vi "Periodic Tasks.vi"(8 "error in":errorcluster) -> ()   [LabVIEW 2016]
doc: "This VI runs in parallel to other tasks. It can contain as many user-defined periodic loops as you need. These can carry out PID or other sorts of timed response."
uses:
  <vilib>/Rock Robotics/WPI/DriverStation/WPI_DriverStationRobotMode2.ctl
  Autonomous VIs/Autonomous Commands/Autonomous Command Names.ctl
  Autonomous VIs/Autonomous Exec/Autonomous Play Definition.ctl
  <vilib>/Rock Robotics/Network Tables/NT Write String Array.vi
  Global Variables/File Path Globals.vi
  Robot Global Data.vi
  <vilib>/Rock Robotics/Network Tables/NT Write String.vi
  Global Variables/Autonomous Exec Info.vi
  <vilib>/Rock Robotics/Network Tables/SD Read String.vi
  Global Variables/Folder Names.vi
  Global Variables/Refnum Names.vi
  <vilib>/Rock Robotics/WPI/Utilities/WPI_GetSetVariantRefNum.vi
  Global Variables/Sensor Data.vi
  Global Variables/Auto Drive Calibrations.vi
panel:
  out "Waveform Chart":T1(graph)
  out "error out":errorcluster
  out "File Name of Play":string
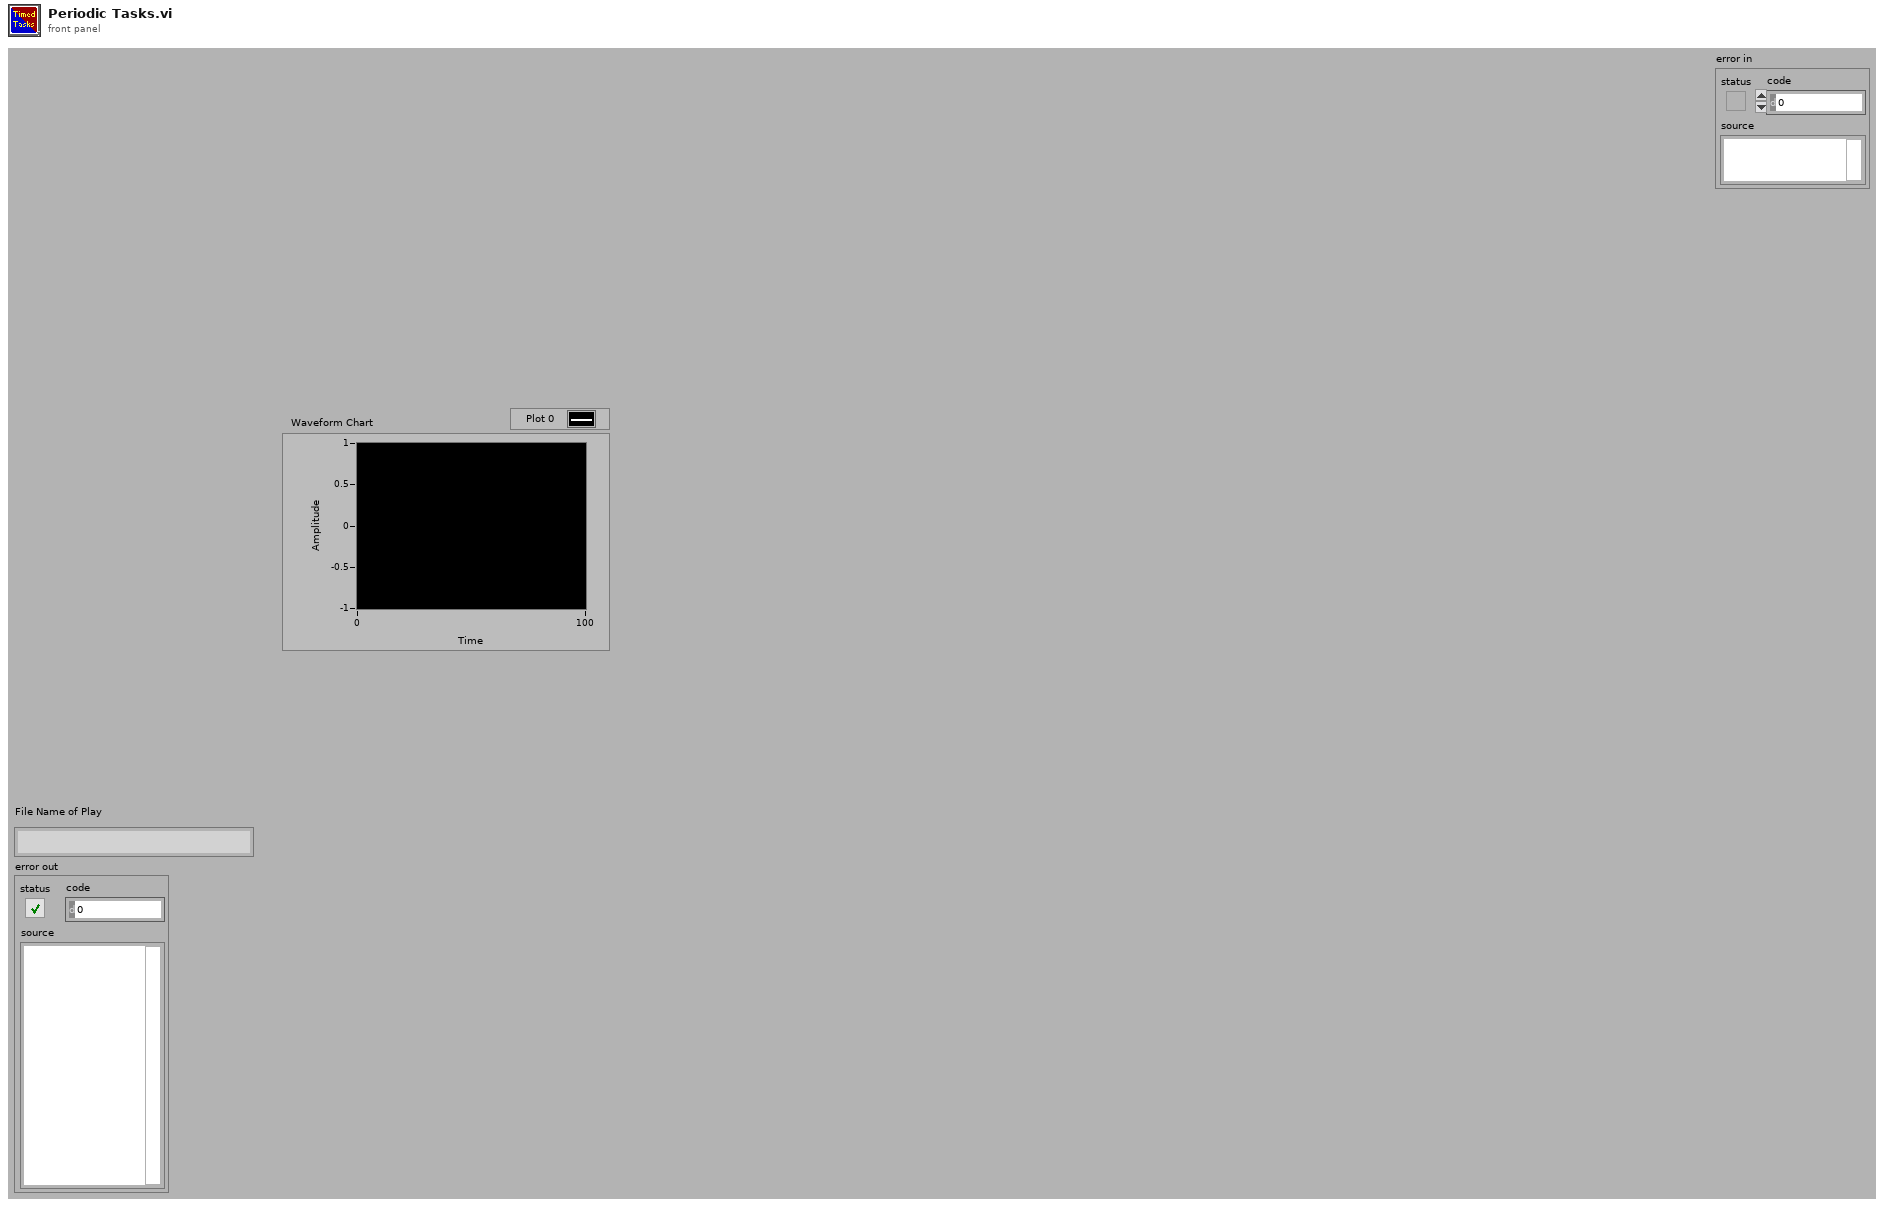
[diagram p1: front panel]
types:
  T1 = cluster{"Goal":dbl, "Process Variable":dbl, "Max Ouput":dbl, dbl, dbl, dbl, dbl}
  T2 = typedef "WPI_DriverStationRobotMode2.ctl" = enum16{"Autonomous Disabled", "Autonomous Enabled", "Teleop Disabled", "Teleop Enabled", "Disconnected", "Finish", "Test Disabled", "Test Enabled", "Emergency Stopped"}
  T3 = typedef "Autonomous Command Names.ctl" = enum16{"No Op", "Command Drive+Climb Shift", "Command Wait", "Command Deliver Gear", "Command Buffer", "Command Drive Path", "Command Drive Time", "Command Shoot", "Command Turn to Heading", "Command Run Conveyor", "Command Spinup Shooter", "Command Deliver Gear Front", "Command Toggle Intake Rotation", "DO NOT USE", "Command Agitate Hopper", "Command Pre-Buffer", "Command Turn to Target", "Command Deliver Gear with Safety", "Command Drive Time with IMU", "Command Drive to Encoders"}
  T4 = typedef "Autonomous Play Definition.ctl" = cluster{"Play Name":string, "Command List":cluster{"Param 1":dbl, "Param 2":dbl, "Autonomous Command Name":T3, "Concurrent":bool, "Param 3":dbl, "Param 4":string}[], "Play Description":string}
  T5 = cluster{"Param 1":dbl, "Param 2":dbl, "Autonomous Command Name":T3, "Concurrent":bool, "Param 3":dbl, "Param 4":string}[]
  T6 = cluster{"Param 1":dbl, "Param 2":dbl, "Autonomous Command Name":T3, "Concurrent":bool, "Param 3":dbl, "Param 4":string}
  T7 = typedef "WPI_JoystickDevRef.ctl" = cluster{"Device":T8}
  T8 = typedef "WPI_JoystickDeviceEnum.ctl" = enum16{"USB 0", "USB 1", "USB 2", "USB 3", "USB 4", "USB 5"}
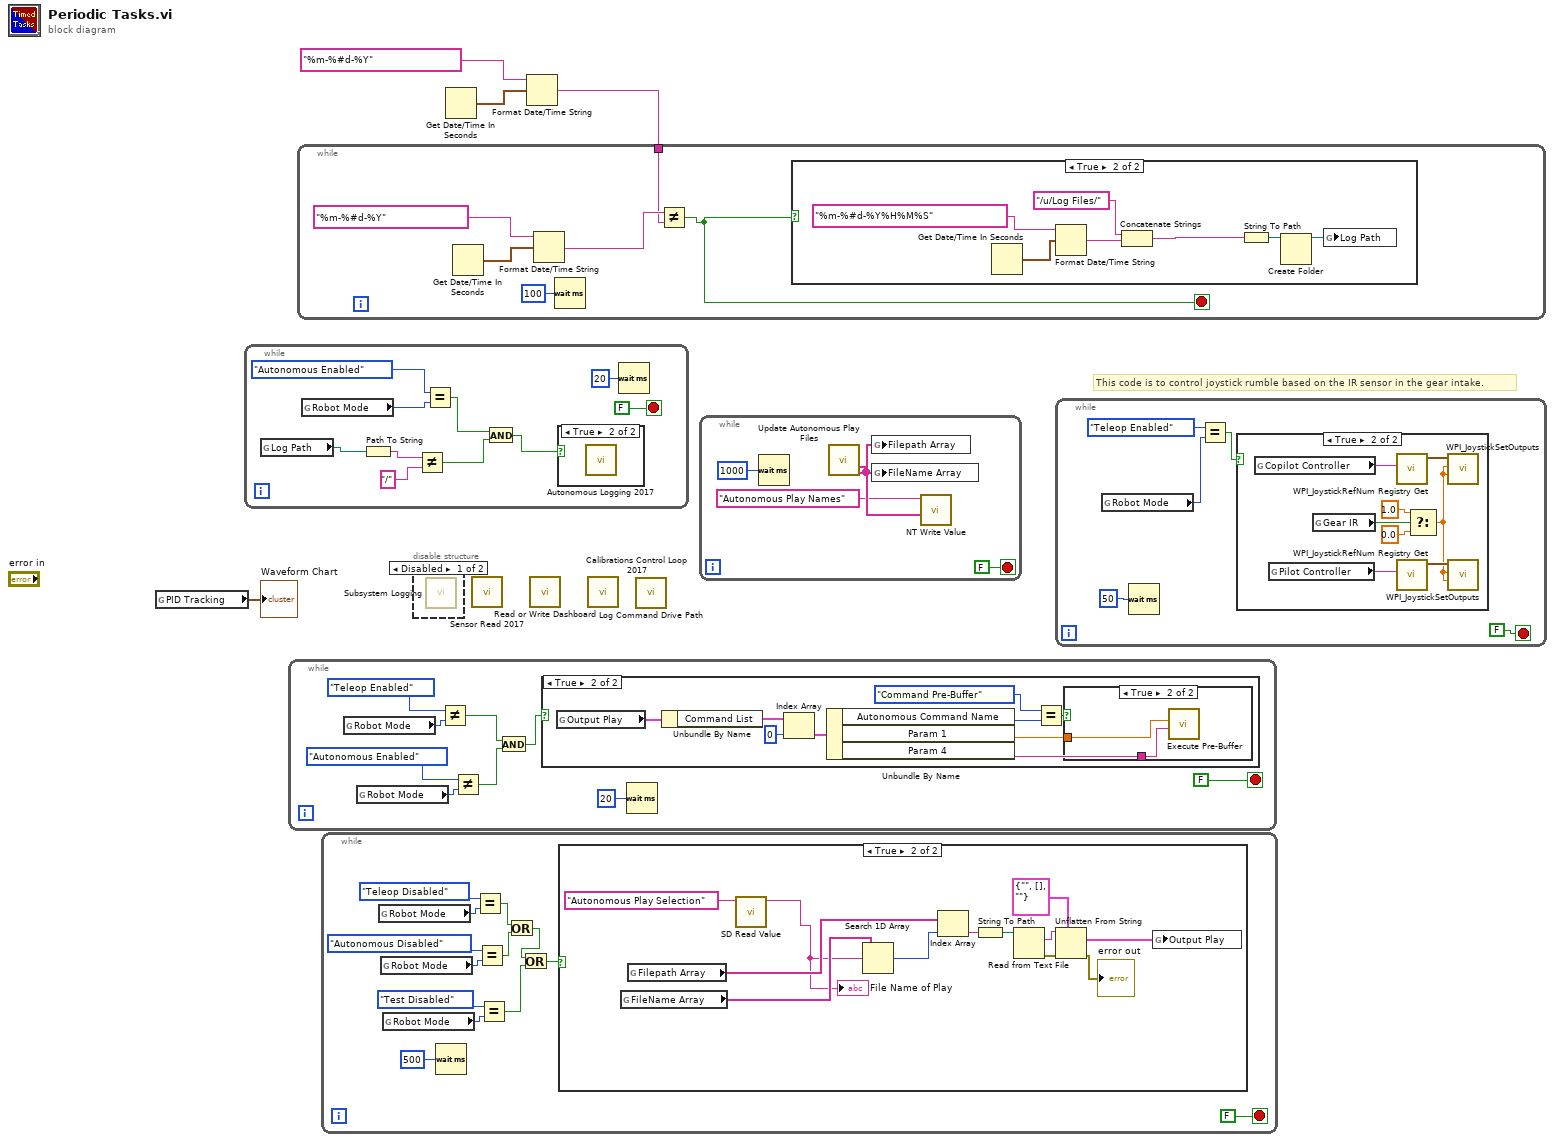
[diagram p0: block diagram]
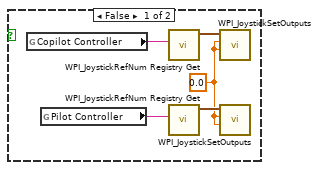
[diagram p3: hidden frame]
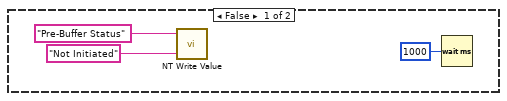
[diagram p7: hidden frame]
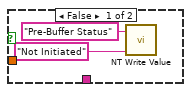
[diagram p8: hidden frame]
diagram:
  # "This code is to control joystick rumble based on the IR sensor in the gear intake."
  n1 = global read "Auto Drive Calibrations.vi" "PID Tracking"() -> (→"Waveform Chart":T1)
  n2 = while {
    stop <- FALSE stop-if-true
    n3 = global read "Folder Names.vi" "Log Path"() -> (w10:path)
    n4 = global read "Robot Global Data.vi" "Robot Mode"() -> (w13:T2)
    n5 = Path To String(path=w10) -> (string=w9:string)
    n6 = Not Equal?(x=w9, y="/") -> (x != y?=w5:bool)
    n7 = Equal?(x=WPI_DriverStationRobotMode2."Autonomous Enabled", y=w13) -> (x = y?=w6:bool)
    n8 = And(x=w6, y=w5) -> (x .and. y?=w7:bool)
    n9 = case shown="True" w7 {
      frame False {
      }
      frame True {
        n10 = call "Autonomous Logging 2017.vi"() -> ()  [unwired: 12 in]
      }
    }
    n11 = Wait (ms)(milliseconds to wait=u32 20) -> ()  [unwired: 1 out]
  }
  n12 = while {
    stop <- FALSE stop-if-true
    n13 = global read "Robot Global Data.vi" "Robot Mode"() -> (w21:T2)
    n14 = global read "Robot Global Data.vi" "Robot Mode"() -> (w19:T2)
    n15 = Not Equal?(x=WPI_DriverStationRobotMode2."Teleop Enabled", y=w21) -> (x != y?=w16:bool)
    n16 = Not Equal?(x=WPI_DriverStationRobotMode2."Autonomous Enabled", y=w19) -> (x != y?=w17:bool)
    n17 = And(x=w16, y=w17) -> (x .and. y?=w15:bool)
    n18 = case shown="True" w15 {
      frame False {
        n19 = call-poly <vilib>:"NT Write Value.vi"("String"="Not Initiated", "Name"="Pre-Buffer Status") -> ()  [unwired: 9 in, 1 out]
        n20 = Wait (ms)(milliseconds to wait=u32 1000) -> ()  [unwired: 1 out]
      }
      frame True {
        n21 = global read "Autonomous Exec Info.vi" "Output Play"() -> (w35:T4)
        n22 = Unbundle By Name(w35) -> ("Command List"=w34:T5)
        n23 = Index Array(array=w34, index=0) -> (element=w32:T6)
        n24 = Unbundle By Name(w32) -> ("Autonomous Command Name"=w31:T3, "Param 1"=w28:dbl, "Param 4"=w27:string)
        n25 = Equal?(x=Autonomous_Command_Names."Command Pre-Buffer", y=w31) -> (x = y?=w29:bool)
        n26 = case shown="True" w29 {
          tunnel: w28 -> [_ w39]
          tunnel: w27 -> [_ w38]
          frame False {
            n27 = call-poly <vilib>:"NT Write Value.vi"("String"="Not Initiated", "Name"="Pre-Buffer Status") -> ()  [unwired: 9 in, 1 out]
          }
          frame True {
            n28 = call "Execute Pre-Buffer.vi"("MP Name"=w38, "PIDF Profile Slot Select"=w39) -> ()  [unwired: 10 in]
          }
        }
      }
    }
    n29 = Wait (ms)(milliseconds to wait=u32 20) -> ()  [unwired: 1 out]
  }
  n30 = while {
    stop <- FALSE stop-if-true
    n31 = global read "Robot Global Data.vi" "Robot Mode"() -> (w51:T2)
    n32 = global read "Robot Global Data.vi" "Robot Mode"() -> (w49:T2)
    n33 = global read "Robot Global Data.vi" "Robot Mode"() -> (w47:T2)
    n34 = Wait (ms)(milliseconds to wait=u32 500) -> ()  [unwired: 1 out]
    n35 = Equal?(x=WPI_DriverStationRobotMode2."Teleop Disabled", y=w51) -> (x = y?=w46:bool)
    n36 = Equal?(x=WPI_DriverStationRobotMode2."Autonomous Disabled", y=w49) -> (x = y?=w45:bool)
    n37 = Equal?(x=WPI_DriverStationRobotMode2."Test Disabled", y=w47) -> (x = y?=w42:bool)
    n38 = Or(x=w46, y=w45) -> (x .or. y?=w43:bool)
    n39 = Or(x=w43, y=w42) -> (x .or. y?=w44:bool)
    n40 = case shown="True" w44 {
      frame False {
      }
      frame True {
        n41 = global read "File Path Globals.vi" "FileName Array"() -> (w64:string[])
        n42 = global read "File Path Globals.vi" "Filepath Array"() -> (w63:string[])
        n43 = call-poly <vilib>:"SD Read Value.vi"("Name"="Autonomous Play Selection") -> ("String"=w55:string)  [unwired: 8 in, 2 out]
        "File Name of Play" <- w55
        n44 = Search 1D Array(1D array=w64, element=w55) -> (index of element=w62:i32)  [unwired: 1 in]
        n45 = Index Array(array=w63, index=w62) -> (element=w61:string)
        n46 = String To Path(string=w61) -> (path=w57:path)
        n47 = Read from Text File(file (use dialog)=w57) -> (text=w60:string, error out=w58:errorcluster)  [unwired: 3 in, 2 out]
        n48 = Unflatten From String(type=T4 {"Play Name"="", "Command List"=[], "Play Description"=""}, binary string=w60, error in (no error)=w58) -> (value=w53:T4, error out=→"error out":errorcluster)  [unwired: 2 in, 1 out]
        n49 = global write "Autonomous Exec Info.vi" "Output Play"(w53) -> ()
      }
    }
  }
  n50 = disable-structure shown="Disabled" {
    frame Disabled {
      n51 = call "Subsystem Logging.vi"() -> ()  [unwired: 12 in]
    }
    frame Enabled {
    }
  }
  n52 = Get Date/Time In Seconds() -> (seconds since 1Jan1904=w3:timestamp)
  n53 = call "Sensor Read 2017.vi"() -> ()  [unwired: 12 in]
  n54 = Format Date/Time String(time format string (%c)="%m-%#d-%Y", seconds (now)=w3) -> (date/time string=w2:string)  [unwired: 1 in]
  n55 = while {
    tunnel: w2 -> [w66]
    stop <- w65 stop-if-true
    n56 = Get Date/Time In Seconds() -> (seconds since 1Jan1904=w70:timestamp)
    n57 = Format Date/Time String(time format string (%c)="%m-%#d-%Y", seconds (now)=w70) -> (date/time string=w67:string)  [unwired: 1 in]
    n58 = Wait (ms)(milliseconds to wait=u32 100) -> ()  [unwired: 1 out]
    n59 = Not Equal?(x=w67, y=w66) -> (x != y?=w65:bool)
    n60 = case shown="True" w65 {
      frame False {
      }
      frame True {
        n61 = Get Date/Time In Seconds() -> (seconds since 1Jan1904=w77:timestamp)
        n62 = Format Date/Time String(time format string (%c)="%m-%#d-%Y%H%M%S", seconds (now)=w77) -> (date/time string=w75:string)  [unwired: 1 in]
        n63 = Concatenate Strings("/u/Log Files/" ("string"), w75) -> (w74:string)
        n64 = String To Path(string=w74) -> (path=w73:path)
        n65 = Create Folder(path (use dialog)=w73) -> (created path=w72:path)  [unwired: 2 in, 2 out]
        n66 = global write "Folder Names.vi" "Log Path"(w72) -> ()
      }
    }
  }
  n67 = call "Read or Write Dashboard.vi"() -> ()  [unwired: 12 in]
  n68 = call "Calibrations Control Loop 2017.vi"() -> ()  [unwired: 12 in]
  n69 = call "Log Command Drive Path.vi"() -> ()  [unwired: 12 in]
  n70 = while {
    stop <- FALSE stop-if-true
    n71 = Wait (ms)(milliseconds to wait=u32 1000) -> ()  [unwired: 1 out]
    n72 = call "Update Autonomous Play Files.vi"() -> ("Filepath Array"=w80:string[], "filename array"=w79:string[])  [unwired: 12 in, 2 out]
    n73 = global write "File Path Globals.vi" "Filepath Array"(w80) -> ()
    n74 = global write "File Path Globals.vi" "FileName Array"(w79) -> ()
    n75 = call-poly <vilib>:"NT Write Value.vi"("String Array"=w79, "Name"="Autonomous Play Names") -> ()  [unwired: 9 in, 1 out]
  }
  n76 = while {
    stop <- FALSE stop-if-true
    n77 = global read "Robot Global Data.vi" "Robot Mode"() -> (w83:T2)
    n78 = Wait (ms)(milliseconds to wait=u32 50) -> ()  [unwired: 1 out]
    n79 = Equal?(x=WPI_DriverStationRobotMode2."Teleop Enabled", y=w83) -> (x = y?=w84:bool)
    n80 = case shown="True" w84 {
      frame False {
        w90 = 0.0
        n81 = global read "Refnum Names.vi" "Copilot Controller"() -> (w88:string)
        n82 = global read "Refnum Names.vi" "Pilot Controller"() -> (w89:string)
        n83 = call <vilib>:"WPI_JoystickRefNum Registry Get.vi"("refnum name"=w88) -> ("JoystickDevRef"=w92:T7)  [unwired: 9 in, 1 out]
        n84 = call <vilib>:"WPI_JoystickRefNum Registry Get.vi"("refnum name"=w89) -> ("JoystickDevRef"=w91:T7)  [unwired: 9 in, 1 out]
        n85 = call <vilib>:"WPI_JoystickSetOutputs.vi"("Right Rumble"=w90, "Left Rumble"=w90, "JoystickDevRef"=w92) -> ()  [unwired: 7 in, 2 out]
        n86 = call <vilib>:"WPI_JoystickSetOutputs.vi"("Right Rumble"=w90, "Left Rumble"=w90, "JoystickDevRef"=w91) -> ()  [unwired: 7 in, 2 out]
      }
      frame True {
        n87 = global read "Refnum Names.vi" "Copilot Controller"() -> (w94:string)
        n88 = global read "Refnum Names.vi" "Pilot Controller"() -> (w95:string)
        n89 = global read "Sensor Data.vi" "Gear IR"() -> (w93:bool)
        n90 = call <vilib>:"WPI_JoystickRefNum Registry Get.vi"("refnum name"=w94) -> ("JoystickDevRef"=w98:T7)  [unwired: 9 in, 1 out]
        n91 = call <vilib>:"WPI_JoystickRefNum Registry Get.vi"("refnum name"=w95) -> ("JoystickDevRef"=w97:T7)  [unwired: 9 in, 1 out]
        n92 = Select(t=1.0, s=w93, f=0.0) -> (s? t:f=w96:dbl)
        n93 = call <vilib>:"WPI_JoystickSetOutputs.vi"("Right Rumble"=w96, "Left Rumble"=w96, "JoystickDevRef"=w98) -> ()  [unwired: 7 in, 2 out]
        n94 = call <vilib>:"WPI_JoystickSetOutputs.vi"("Right Rumble"=w96, "Left Rumble"=w96, "JoystickDevRef"=w97) -> ()  [unwired: 7 in, 2 out]
      }
    }
  }
